vi "CLAD Exercise 3-7.vi"() -> ()   [LabVIEW 2014]
panel:
  out "Numeric 2":dbl
  in  "Numeric":dbl
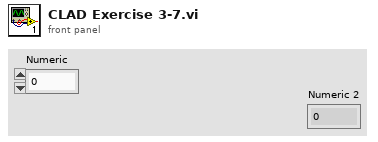
[diagram p1: front panel]
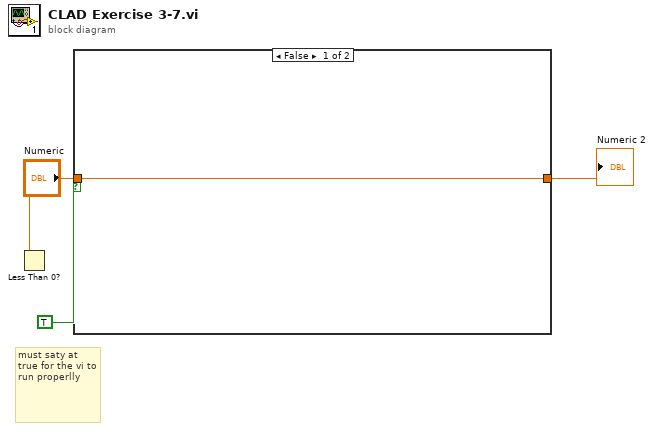
[diagram p0: block diagram]
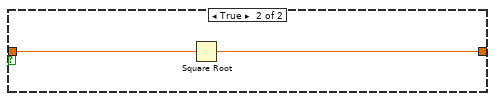
[diagram p2: hidden frame]
diagram:
  # "must saty at true for the vi to run properlly"
  n1 = Less Than 0?(x="Numeric") -> ()  [unwired: 1 out]
  n2 = case shown="False" TRUE {
    tunnel: "Numeric" -> [w4 w6]
    tunnel: [w4 w5] -> w2
    frame False {
    }
    frame True {
      n3 = Square Root(x=w6) -> (sqrt(x)=w5:dbl)
    }
  }
  "Numeric 2" <- w2
